vi "lut_2d.vi"() -> (0 "output array":dbl[][](array[numeric])=[[3.927, 4.248, 4.712, 5.176, 5.498], [3.605, 3.927, 4.712, 5.498, 5.82], [3.142, 3.142, nan, 0.0, 0.0], [2.678, 2.356, 1.571, 0.785, 0.464], [2.356, 2.034, 1.571, 1.107, 0.785]])   [LabVIEW 2015, in "PolyVIEW.lvclass"]
uses:
  PolyVIEW.lvclass
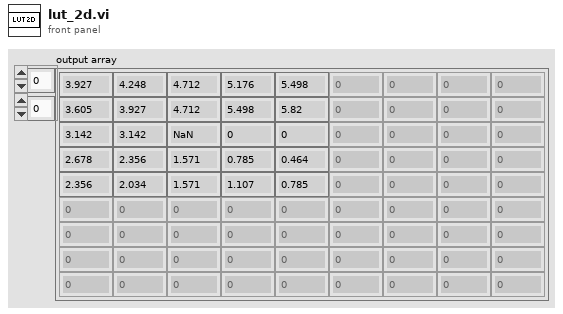
[diagram p1: front panel]
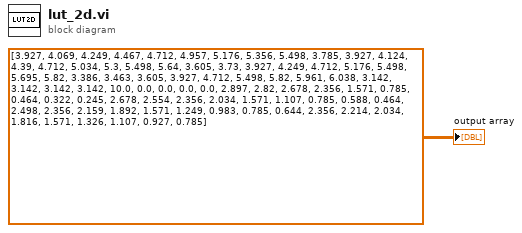
[diagram p0: block diagram]
diagram:
  "output array" <- dbl[][] [[3.927, 4.069, 4.249, 4.467, 4.712, 4.957, 5.176, 5.356, 5.498], [3.785, 3.927, 4.124, 4.39, 4.712, 5.034, 5.3, 5.498, 5.64], [3.605, 3.73, 3.927, 4.249, 4.712, 5.176, 5.498, 5.695, 5.82], [3.386, 3.463, 3.605, 3.927, 4.712, 5.498, 5.82, 5.961, 6.038], [3.142, 3.142, 3.142, 3.142, 10.0, 0.0, 0.0, 0.0, 0.0], [2.897, 2.82, 2.678, 2.356, 1.571, 0.785, 0.464, 0.322, 0.245], [2.678, 2.554, 2.356, 2.034, 1.571, 1.107, 0.785, 0.588, 0.464], [2.498, 2.356, 2.159, 1.892, 1.571, 1.249, 0.983, 0.785, 0.644], [2.356, 2.214, 2.034, 1.816, 1.571, 1.326, 1.107, 0.927, 0.785]] ("output array")
